vi "Timer.vi"(8 "error in (no error)":errorcluster, 10 "Target Time":i32, 11 "Timer Command":T1) -> (0 "error out":errorcluster, 2 "Done?":bool=TRUE, 3 "Elapsed Time":dbl)   [LabVIEW 2013]
uses:
  Timer Command Control.ctl
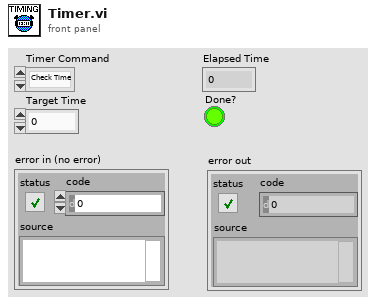
[diagram p1: front panel]
types:
  T1 = typedef "Timer Command Control.ctl" = enum16{"Check Time", "Set Time"}
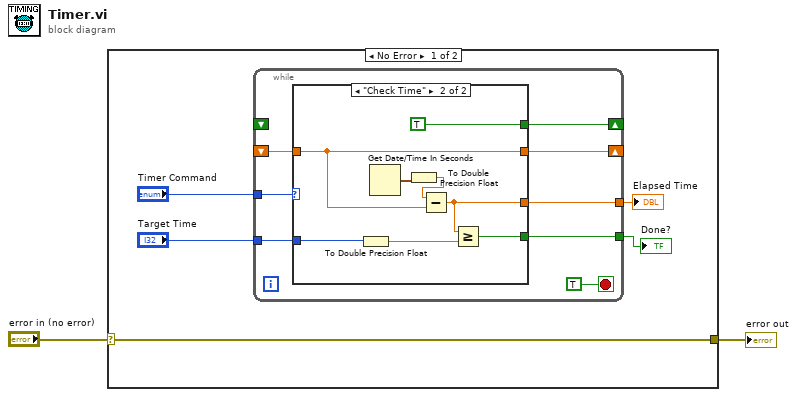
[diagram p0: block diagram]
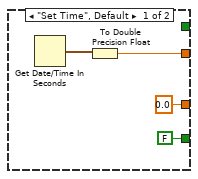
[diagram p2: hidden frame]
diagram:
  n1 = case shown="No Error" "error in (no error)" {
    selector: "error in (no error)" -> [w3 w28]
    tunnel: [w3 w28] -> w2
    frame No Error {
      n2 = while {
        shift-right: [w15] -> _
        shift-left: _ -> [w12]
        tunnel: "Timer Command" -> [w14]
        tunnel: "Target Time" -> [w13]
        tunnel: [w11] -> w5
        tunnel: [w10] -> w4
        shift-right: [w8] -> _
        shift-left: _ -> [_]
        stop <- TRUE stop-if-true
        n3 = case shown="\"Check Time\"" w14 {
          tunnel: [w18 w27] -> w15
          tunnel: w13 -> [_ w24]
          tunnel: w12 -> [_ w27]
          tunnel: [0.0 w23] -> w11
          tunnel: [FALSE w21] -> w10
          tunnel: [_ TRUE] -> w8
          frame "Set Time", Default {
            n4 = Get Date/Time In Seconds() -> (seconds since 1Jan1904=w19:timestamp)
            n5 = To Double Precision Float(number=w19) -> (double precision float=w18:dbl)
          }
          frame "Check Time" {
            n6 = To Double Precision Float(number=w24) -> (double precision float=w22:dbl)
            n7 = Get Date/Time In Seconds() -> (seconds since 1Jan1904=w26:timestamp)
            n8 = To Double Precision Float(number=w26) -> (double precision float=w25:dbl)
            n9 = Subtract(x=w25, y=w27) -> (x-y=w23:dbl)
            n10 = Greater Or Equal?(x=w23, y=w22) -> (x >= y?=w21:bool)
          }
        }
      }
      "Elapsed Time" <- w5
      "Done?" <- w4
    }
    frame Error {
    }
  }
  "error out" <- w2
